vi "Query Chan Parameters (Mode).vi"(7 "Channel (1: Chan A)":i32(ring)=1 items=["Channel A"=1, "Channel B"=2, "Channel C"=3, "Channel D"=4, "Channel E"=5, "Channel F"=6, "Channel G"=7, "Channel H"=8], 8 "error in (no error)":errorcluster, 11 "VISA resource name":refnum<visa-resource-name>) -> (0 "error out":errorcluster, 2 "Mode Parameters":T1={"Mode"=enum."Normal", "Burst #"=-1, "DC Off"=-1, "DC On"=-1, "Delay"=nan, "Width"=nan, "Wait #"=-1} {"Width" format="%.3p"; "Delay" format="%.3p"}, 3 "VISA resource name out":refnum<visa-resource-name>)   [LabVIEW 2012, in "Berkeley Nucleonics 500 Series.lvlib"]
doc: "This VI is used to read the mode configuration of the selected channel."
uses:
  Berkeley Nucleonics 500 Series.lvlib
panel:
  # "Normal\nSingle\nBurst"
  # "Burst"
  # "Duty\nCycle"
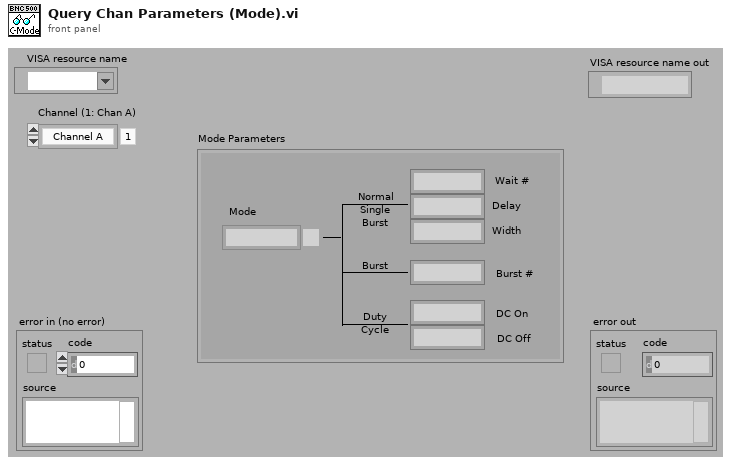
[diagram p1: front panel]
types:
  T1 = cluster{"Mode":enum16{"Normal", "Single", "Burst", "Duty Cycle"}, "Burst #":i32, "DC Off":i32, "DC On":i32, "Delay":dbl, "Width":dbl, "Wait #":i32}
  T2 = cluster{"Chan Mode":enum16{"Normal", "Single", "Burst", "Duty Cycle"}, "Chan Burst #":i32, "Chan DC Off":i32, "Chan DC On":i32, "Chan Delay":dbl, "Chan Width":dbl, "Chan Wait #":i32}
  T3 = enum16{"Normal", "Single", "Burst", "Duty Cycle"}
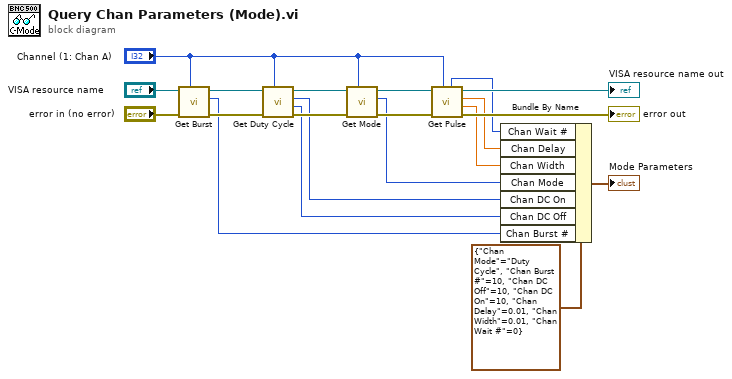
[diagram p0: block diagram]
diagram:
  n1 = call "Get Burst.vi"("Channel (1: Chan A)"="Channel (1: Chan A)", "error in (no error)"="error in (no error)", "VISA resource name"="VISA resource name") -> ("error out"=w10:errorcluster, "Burst #"=w6:i32, "VISA resource name out"=w11:refnum<visa-resource-name>)  [unwired: 6 out]
  n2 = call "Get Duty Cycle.vi"("Channel (1: Chan A)"="Channel (1: Chan A)", "error in (no error)"=w10, "VISA resource name"=w11) -> ("error out"=w13:errorcluster, "DC Off"=w5:i32, "DC On"=w4:i32, "VISA resource name out"=w12:refnum<visa-resource-name>)  [unwired: 5 out]
  n3 = call "Get Mode.vi"("Channel (1: Chan A)"="Channel (1: Chan A)", "error in (no error)"=w13, "VISA resource name"=w12) -> ("error out"=w14:errorcluster, "Mode"=w7:T3, "VISA resource name out"=w15:refnum<visa-resource-name>)  [unwired: 6 out]
  n4 = call "Get Pulse.vi"("Channel (1: Chan A)"="Channel (1: Chan A)", "error in (no error)"=w14, "VISA resource name"=w15) -> ("error out"=→"error out":errorcluster, "Width"=w3:dbl, "Delay"=w2:dbl, "VISA resource name out"=→"VISA resource name out":refnum<visa-resource-name>, "Wait #"=w1:i32)  [unwired: 4 out]
  n5 = Bundle By Name(cluster=T2 {"Chan Mode"=enum."Duty Cycle", "Chan Burst #"=10, "Chan DC Off"=10, "Chan DC On"=10, "Chan Delay"=0.01, "Chan Width"=0.01, "Chan Wait #"=0} ("Mode Parameters"), "Chan Wait #"=w1, "Chan Delay"=w2, "Chan Width"=w3, "Chan Mode"=w7, "Chan DC On"=w4, "Chan DC Off"=w5, "Chan Burst #"=w6) -> (→"Mode Parameters":T2)
